vi "(Sub) Run Loop.vi"(8 "error in (no error)":errorcluster caption="에러 입력(에러 없음)") -> (0 "error out":errorcluster caption="에러 출력")   [LabVIEW 2017]
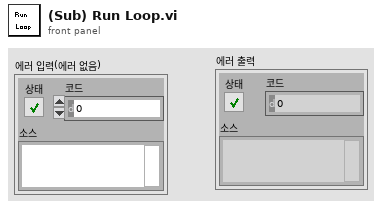
[diagram p1: front panel]
types:
  T1 = enum32{"Bad", "Idle", "Run top level", "Running"}
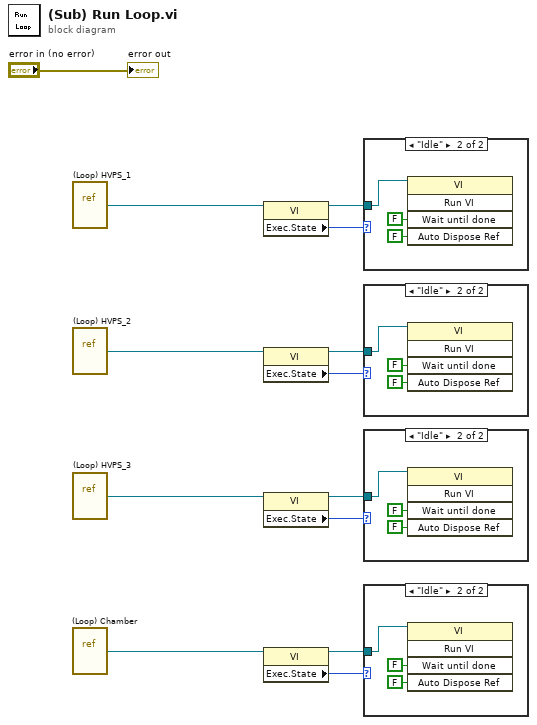
[diagram p0: block diagram]
diagram:
  n1 = vi-ref "(Loop) HVPS_1.vi"() -> (w13:refnum<vi>)
  n2 = vi-ref "(Loop) HVPS_2.vi"() -> (w8:refnum<vi>)
  n3 = vi-ref "(Loop) HVPS_3.vi"() -> (w7:refnum<vi>)
  n4 = vi-ref "(Loop) Chamber.vi"() -> (w1:refnum<vi>)
  n5 = property class="VI"(reference=w13) -> (reference out=w11:refnum<vi>, "Exec.State"=w12:T1)  [unwired: 1 in, 1 out]
  n6 = property class="VI"(reference=w8) -> (reference out=w10:refnum<vi>, "Exec.State"=w9:T1)  [unwired: 1 in, 1 out]
  n7 = property class="VI"(reference=w7) -> (reference out=w5:refnum<vi>, "Exec.State"=w6:T1)  [unwired: 1 in, 1 out]
  n8 = property class="VI"(reference=w1) -> (reference out=w3:refnum<vi>, "Exec.State"=w2:T1)  [unwired: 1 in, 1 out]
  n9 = case shown="\"Idle\"" w12 {
    tunnel: w11 -> [_ w16]
    frame "Bad", Default {
    }
    frame "Idle" {
      n10 = invoke class="VI" method="Run VI"(reference=w16, "Wait until done"=FALSE ("완료될 때까지 기다림"), "Auto Dispose Ref"=FALSE ("참조 자동 삭제")) -> ()  [unwired: 2 in, 5 out]
    }
  }
  n11 = case shown="\"Idle\"" w9 {
    tunnel: w10 -> [_ w19]
    frame "Bad", Default {
    }
    frame "Idle" {
      n12 = invoke class="VI" method="Run VI"(reference=w19, "Wait until done"=FALSE ("완료될 때까지 기다림"), "Auto Dispose Ref"=FALSE ("참조 자동 삭제")) -> ()  [unwired: 2 in, 5 out]
    }
  }
  n13 = case shown="\"Idle\"" w6 {
    tunnel: w5 -> [_ w22]
    frame "Bad", Default {
    }
    frame "Idle" {
      n14 = invoke class="VI" method="Run VI"(reference=w22, "Wait until done"=FALSE ("완료될 때까지 기다림"), "Auto Dispose Ref"=FALSE ("참조 자동 삭제")) -> ()  [unwired: 2 in, 5 out]
    }
  }
  n15 = case shown="\"Idle\"" w2 {
    tunnel: w3 -> [_ w25]
    frame "Bad", Default {
    }
    frame "Idle" {
      n16 = invoke class="VI" method="Run VI"(reference=w25, "Wait until done"=FALSE ("완료될 때까지 기다림"), "Auto Dispose Ref"=FALSE ("참조 자동 삭제")) -> ()  [unwired: 2 in, 5 out]
    }
  }
  "error out" <- "error in (no error)"
